vi "_Test Abort Running Test.vi"(8 "error in (no error)":errorcluster, 11 "Abort Test in":refnum<class "Abort Test.lvclass">) -> (0 "error out":errorcluster, 3 "Abort Test out":refnum<class "Abort Test.lvclass">)   [LabVIEW 2020, in "LUnit Tests.lvlib" / "Abort Test.lvclass"]
uses:
  Abort Test.lvclass
  source/Framework/Execution API/Execution API.lvclass
  Test Dummys/Hanging Dummy Case/Hanging Dummy Case.lvclass
  <vilib>/Astemes/LUnit/Test Case.lvclass
  C:/Git/astemes-lunit/source/Framework/Test Case/LUnit Test Case.lvclass
  C:/Git/astemes-lunit/tests/Test Dummys/Hanging Dummy Case/Hanging Dummy Case.lvclass
  C:/Program Files (x86)/National Instruments/LabVIEW 2021/vi.lib/Astemes/LUnit/Test Case.lvclass
  C:/Git/astemes-lunit/tests/Abort Test/Abort Test.lvclass
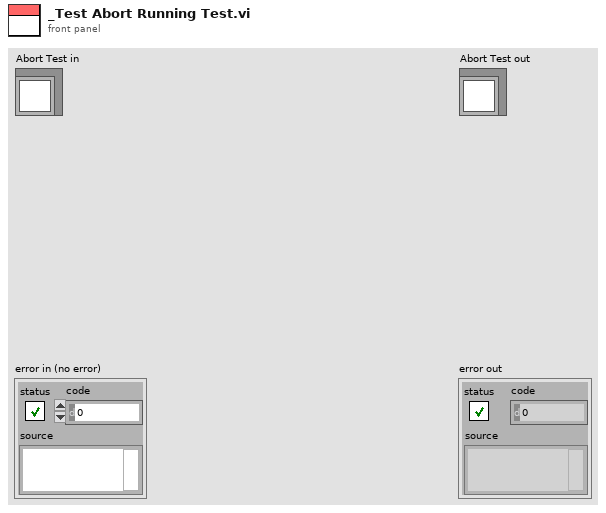
[diagram p1: front panel]
types:
  T1 = cluster{"Result Events":refnum<event-registration>, "Event Registration Refnum":refnum<event-registration>}
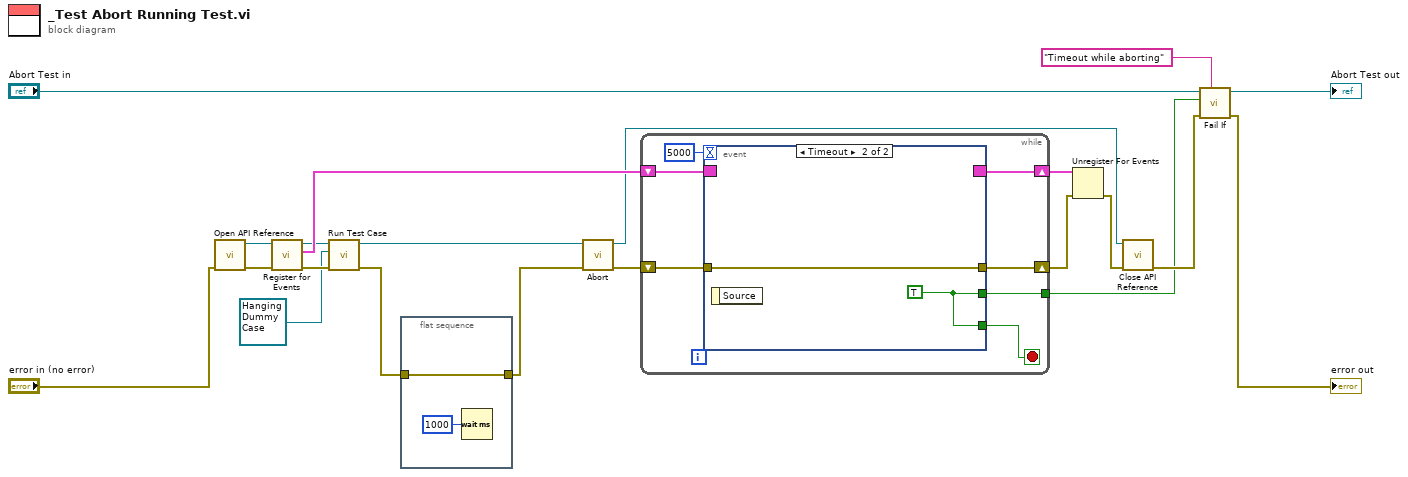
[diagram p0: block diagram]
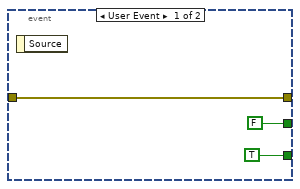
[diagram p2: hidden frame]
diagram:
  n1 = call "Open API Reference.vi"("error in (no error)"="error in (no error)") -> ("error out"=w15:errorcluster, "Execution API out"=w14:refnum<class "Execution API.lvclass">)  [unwired: 9 in]
  n2 = call "Register for Events.vi"("error in (no error)"=w15, "Execution API in"=w14) -> ("error out"=w17:errorcluster, "Event Registrations"=w18:T1, "Execution API out"=w16:refnum<class "Execution API.lvclass">)  [unwired: 7 in]
  n3 = call "Run Test Case.vi"("error in (no error)"=w17, "Test Case"=refnum<class "Hanging Dummy Case.lvclass"> refnum ("Hanging Demo Case.lvclass"), "Execution API In"=w16) -> ("error out"=w1:errorcluster, "Execution API Out"=w5:refnum<class "Execution API.lvclass">)  [unwired: 7 in]
  n4 = flat-sequence {
    tunnel: [w23] -> w2
    tunnel: w1 -> [w23]
    frame #0 {
      n5 = Wait (ms)(milliseconds to wait=u32 1000) -> ()  [unwired: 1 out]
    }
  }
  n6 = call "Abort.vi"("error in (no error)"=w2, "Execution API in"=w5) -> ("error out"=w3:errorcluster, "Execution API out"=w4:refnum<class "Execution API.lvclass">)  [unwired: 8 in]
  n7 = while {
    shift-right: [w29] -> w19
    shift-left: w18 -> [w30]
    shift-right: [w27] -> w20
    shift-left: w3 -> [w28]
    tunnel: [w25] -> w6
    stop <- w24 stop-if-true
    n8 = event shown="[1] Timeout" {
      selector: w30 -> [_ _]
      dyn-events: [_ _] -> w29
      timeout: 5000 -> [_ _]
      tunnel: w28 -> [w33 w35]
      tunnel: [w33 w35] -> w27
      tunnel: [FALSE w34] -> w25
      tunnel: [TRUE w34] -> w24
      event User Event {
        n9 = event-data() -> ()  [unwired: 1 in, 1 out]
      }
      event Timeout {
        w34 = TRUE
        n10 = event-data() -> ()  [unwired: 1 in, 1 out]
      }
    }
  }
  n11 = Unregister For Events(event registration refnum=w19, error in=w20) -> (error out=w21:errorcluster)
  n12 = call "Close API Reference.vi"("error in (no error)"=w21, "Execution API in"=w4) -> ("error out"=w8:errorcluster)  [unwired: 9 in]
  n13 = call <vilib>:"Fail If.vi"("Description"="Timeout while aborting", "error in (no error)"=w8, "Fail?"=w6, "LUnit Test Case In"="Abort Test in") -> ("error out"=→"error out":errorcluster, "LUnit Test Case Out"=→"Abort Test out":refnum<class "Abort Test.lvclass">)  [unwired: 6 in]
